vi "Read Durations.vi"(8 "error in (no error)":errorcluster, 11 "Framework Performance in":refnum<class "Performance.lvclass">) -> (0 "error out":errorcluster, 1 "tx duration":u32 format="%d us", 2 "rx duration":u32 format="%d us", 3 "Framework Performance out":refnum<class "Performance.lvclass">)   [LabVIEW 2017, in "DSF Core.lvlib" / "Performance.lvclass"]
uses:
  Performance.lvclass
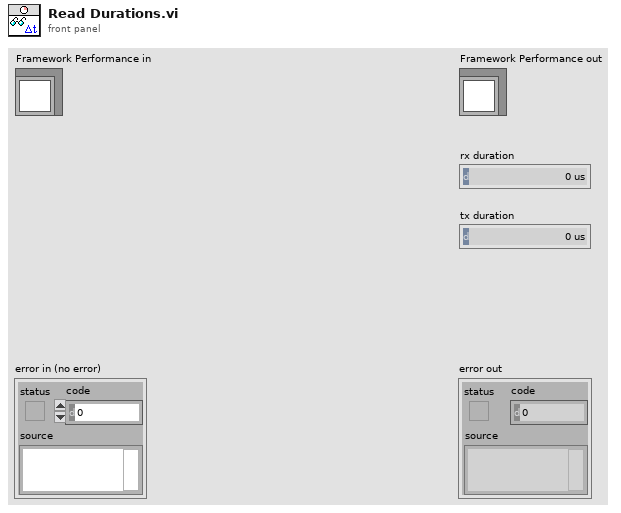
[diagram p1: front panel]
types:
  T1 = typedef "DSF Core.lvlib/Timing Status Pointer.lvclass/Timing Status Data.ctl" = cluster{"rx start time":u32, "rx end time":u32, "tx start time":u32, "tx end time":u32, "cycle start time":u32, "cycle end time":u32, "prev start time":u32}
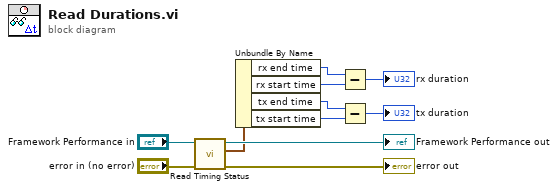
[diagram p0: block diagram]
diagram:
  n1 = call "Read Timing Status.vi"("error in (no error)"="error in (no error)", "Framework Performance in"="Framework Performance in") -> ("error out"=→"error out":errorcluster, "timing status"=w5:T1, "Framework Performance out"=→"Framework Performance out":refnum<class "Performance.lvclass">)  [unwired: 7 in]
  n2 = Unbundle By Name(w5) -> ("rx end time"=w11:u32, "rx start time"=w10:u32, "tx end time"=w2:u32, "tx start time"=w3:u32)
  n3 = Subtract(x=w11, y=w10) -> (x-y=→"rx duration":u32)
  n4 = Subtract(x=w2, y=w3) -> (x-y=→"tx duration":u32)
